vi "Find active route.vi"(8 "error in":errorcluster, 11 "2525 in":refnum<class "2525.lvclass">) -> (0 "error out":errorcluster, 2 "Active Route":string[](array[string]), 3 "2525 out":refnum<class "2525.lvclass">)   [LabVIEW 2019, in "2525.lvlib" / "2525.lvclass"]
uses:
  Library/2525.lvclass
  Library/2525.lvclass/2525.ctl
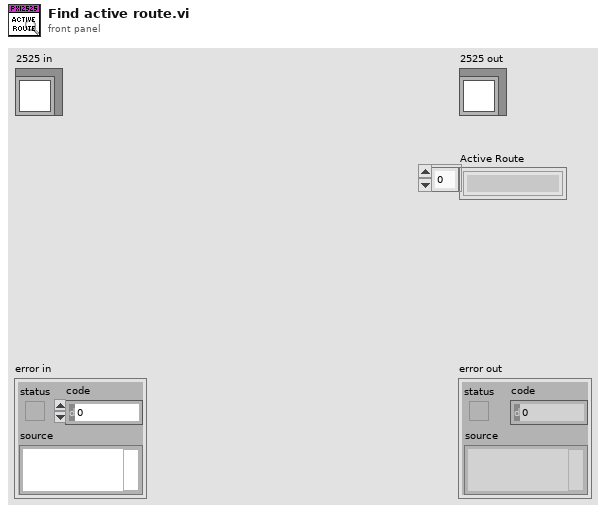
[diagram p1: front panel]
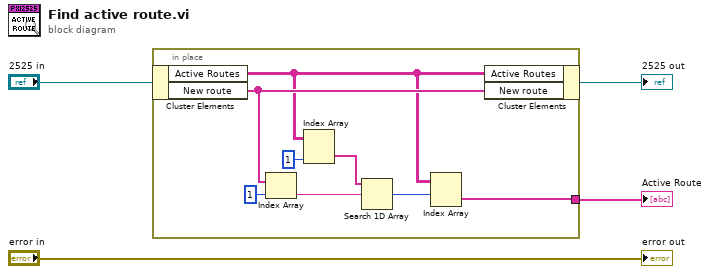
[diagram p0: block diagram]
diagram:
  n1 = in-place {
    in-place-border: [w5] -> w1
    n2 = in-place-cluster #1("2525 in") -> ("Active Routes"=w6:string[][], "New route"=w12:string[])
    n3 = Index Array(array=w12, index=1) -> (element=w10:string)
    n4 = Index Array(array=w6, index (col)=1 ("disabled index (col)")) -> (element=w11:string[])  [unwired: 1 in]
    n5 = Search 1D Array(1D array=w11, element=w10) -> (index of element=w7:i32)  [unwired: 1 in]
    n6 = Index Array(array=w6, index (row)=w7) -> (element=w5:string[])  [unwired: 1 in]
    n7 = in-place-cluster #1("Active Routes"=w6, "New route"=w12) -> (→"2525 out":refnum<class "2525.lvclass">)
  }
  "Active Route" <- w1
  "error out" <- "error in"
